vi "AlliGator Get Series Subfolders Information.vi"(8 "error in (no error)":errorcluster, 10 "pattern":string, 11 "Path":path) -> (0 "error out":errorcluster, 1 "Subfolder Paths":path[](array[path]), 2 "Sorted Subfolder Names":string[](array[string]), 3 "dup directory path":path, 4 "# Files":i32[](array[numeric]), 5 "Files in the Root Folder":string[](array[string]), 6 "Same # Files?":bool)   [LabVIEW 2021, in "AlliGator Scripts.lvlib"]
doc: "Returns a breadown of the folder's content for subsequent script actions."
uses:
  AlliGator Scripts.lvlib
  <userlib>/_OpenG.lib/file/file.llb/openg_file.lvlib
  Strings/Strings.lvlib
panel:
  # "see the AlliGator License on the block diagram (Ctrl+E or Window:Show Block Diagram)"
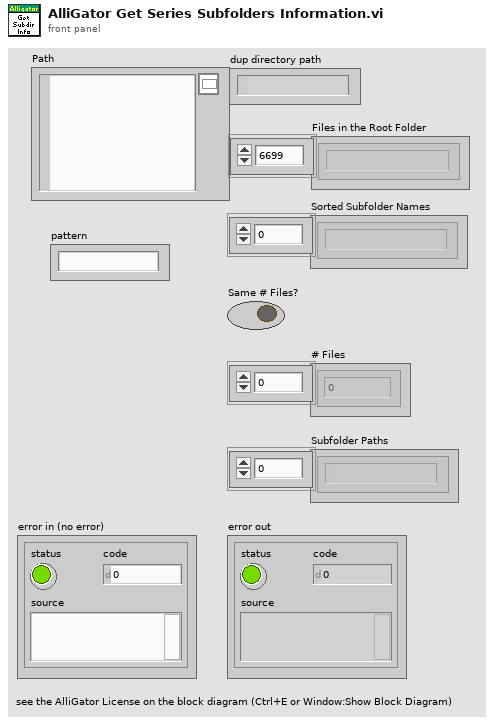
[diagram p1: front panel]
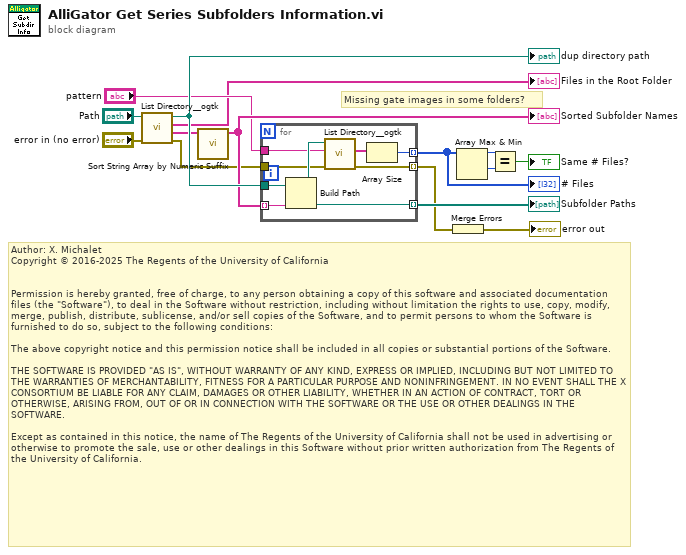
[diagram p0: block diagram]
diagram:
  # "Author: X. Michalet\nCopyright © 2016-2025 The Regents of the University of California\n \n\nPermission is hereby granted, free of charge, to any person obtaining a copy of this software and associated documentation files (the \"Software\"), to deal in the Software without restriction, including without limitation the rights to use, copy, modify, merge, publish, distribute, sublicense, and/or sell copies of the Software, and to permit persons to whom the Software is furnished to do so, subject to the following conditions:\n\nThe above copyright notice and this permission notice shall be included in all copies or substantial portions of the Software.\n\nTHE SOFTWARE IS PROVIDED \"AS IS\", WITHOUT WARRANTY OF ANY KIND, EXPRESS OR IMPLIED, INCLUDING BUT NOT LIMITED TO THE WARRANTIES OF MERCHANTABILITY, FITNESS FOR A PARTICULAR PURPOSE AND NONINFRINGEMENT. IN NO EVENT SHALL THE X CONSORTIUM BE LIABLE FOR ANY CLAIM, DAMAGES OR OTHER LIABILITY, WHETHER IN AN ACTION OF CONTRACT, TORT OR OTHERWISE, ARISING FROM, OUT OF OR IN CONNECTION WITH THE SOFTWARE OR THE USE OR OTHER DEALINGS IN THE SOFTWARE.\n\nExcept as contained in this notice, the name of The Regents of the University of California shall not be used in advertising or otherwise to promote the sale, use or other dealings in this Software without prior written authorization from The Regents of the University of California."
  # "Missing gate images in some folders?"
  n1 = call <userlib>:"List Directory__ogtk.vi"("error in (no error)"="error in (no error)", "directory path"="Path") -> ("error out"=w3:errorcluster, "directory names"=w13:string[], "file names"=→"Files in the Root Folder":string[], "dup directory path"=w15:path)  [unwired: 2 in]
  "dup directory path" <- w15
  n2 = call "Sort String Array by Numeric Suffix.vi"("String Array"=w13) -> ("Sorted String Array"=w14:string[])  [unwired: 8 in, 2 out]
  "Sorted Subfolder Names" <- w14
  n3 = for {
    tunnel: w14 -> [w23] mode=indexing
    tunnel: w15 -> [w22]
    tunnel: [w20] -> w4 mode=indexing
    tunnel: [w19] -> w12 mode=indexing
    tunnel: "pattern" -> [w18]
    tunnel: w3 -> [w17]
    tunnel: [w16] -> w2 mode=indexing
    n4 = Build Path(base path=w22, name or relative path=w23) -> (appended path=w20:path)
    n5 = call <userlib>:"List Directory__ogtk.vi"("error in (no error)"=w17, "pattern"=w18, "directory path"=w20) -> ("error out"=w16:errorcluster, "file names"=w21:string[])  [unwired: 1 in, 2 out]
    n6 = Array Size(array=w21) -> (size(s)=w19:i32)
  }
  "# Files" <- w12
  "Subfolder Paths" <- w4
  n7 = Merge Errors(w2) -> (→"error out":errorcluster)
  n8 = Array Max & Min(array=w12) -> (max value=w8:i32, min value=w6:i32)  [unwired: 2 out]
  n9 = Equal?(x=w8, y=w6) -> (x = y?=→"Same # Files?":bool)
